vi "Get Point Data.vi"(10 "Point Ident":string, 11 "Task Actor in":refnum<class "Task Actor.lvclass">) -> (1 "found?":bool, 2 "value":variant, 3 "Task Actor out":refnum<class "Task Actor.lvclass">)   [LabVIEW 2023, in "Task Actor.lvlib" / "Task Actor.lvclass"]
uses:
  Task Actor.lvclass
  Task Actor.lvclass/Task Actor.ctl
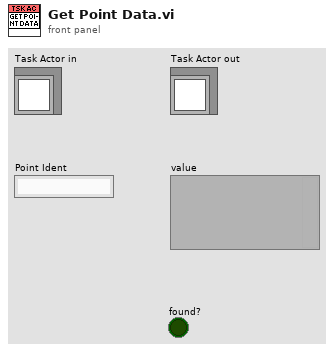
[diagram p1: front panel]
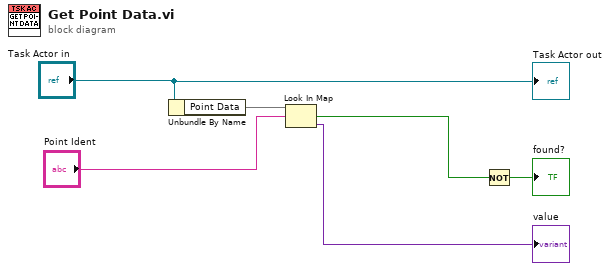
[diagram p0: block diagram]
diagram:
  n1 = Unbundle By Name("Task Actor in") -> ("Point Data"=w5:map{string, variant})
  n2 = Look In Map(map=w5, key="Point Ident") -> (key not found?=w3:bool, value=→"value":variant)  [unwired: 1 in]
  n3 = Not(x=w3) -> (.not. x?=→"found?":bool)
  "Task Actor out" <- "Task Actor in"
